vi "Create Database.vi"(8 "error in (no error)":errorcluster caption="entrée d'erreur (pas d'erreur)", 11 "Database Drivers en entrée":refnum<class "Database Drivers.lvclass">) -> (0 "error out":errorcluster caption="sortie d'erreur", 3 "Database Drivers en sortie":refnum<class "Database Drivers.lvclass">)   [LabVIEW 2020, in "Library Instrument & Equipement.lvlib" / "Library Database.lvlib" / "Database Drivers.lvclass"]
uses:
  Database Drivers.lvclass
  <vilib>/addons/database/Command.llb/Cmd Execute.vi
  <vilib>/addons/database/Recordset.llb/Rec Destroy - Command.vi
  <vilib>/addons/database/Command.llb/Cmd Delete.vi
  Database Drivers.lvclass/Database Drivers.ctl
  <vilib>/addons/database/NI_Database_API.lvlib
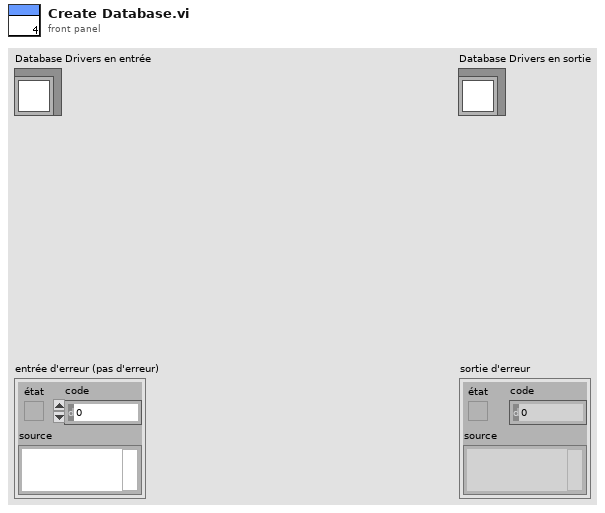
[diagram p1: front panel]
types:
  T1 = typedef "NI_Database_API.lvlib/Conn ObjectReference.ctl" = refnum<k1>
  T2 = typedef "NI_Database_API.lvlib/Cmd ObjectReference.ctl" = refnum<k1>
  T3 = typedef "NI_Database_API.lvlib/Cmd-Rec Object Reference.ctl" = refnum<k1>
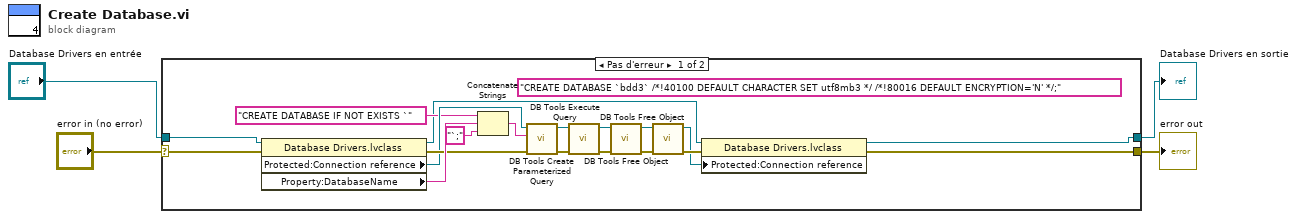
[diagram p0: block diagram]
diagram:
  n1 = case shown="Pas d'erreur" "error in (no error)" {
    selector: "error in (no error)" -> [w22 w25]
    tunnel: [w6 w25] -> w3
    tunnel: [w7 w24] -> w1
    tunnel: "Database Drivers en entrée" -> [w23 w24]
    frame No Error {
      (unwired) "CREATE DATABASE `bdd3` /*!40100 DEFAULT CHARACTER SET utf8mb3 */ /*!80016 DEFAULT ENCRYPTION='N' */;"
      n2 = property class="Database Drivers.lvclass"(reference=w23, error in=w22) -> (reference out=w8:refnum<class "Database Drivers.lvclass">, error out=w14:errorcluster, "Protected:Connection reference"=w11:T1, "Property:DatabaseName"=w16:string)
      n3 = Concatenate Strings("CREATE DATABASE IF NOT EXISTS `" ("chaîne"), w16, "`;" ("chaîne")) -> (w15:string)
      n4 = call <vilib>:"DB Tools Create Parameterized Query.vi"("error in (no error)"=w14, "SQL query"=w15, "connection reference"=w11) -> ("error out"=w21:errorcluster, "command reference"=w20:T2)  [unwired: 4 in, 1 out]
      n5 = call-poly <vilib>:"DB Tools Execute Query.vi"("error in (no error)"=w21, "command reference"=w20) -> ("error out"=w13:errorcluster, "command-recordset reference"=w18:T3)  [unwired: 6 in]
      n6 = call-poly <vilib>:"DB Tools Free Object.vi"("error in (no error)"=w13, "command-recordset reference"=w18) -> ("error out"=w12:errorcluster, "command reference"=w19:T2)  [unwired: 8 in]
      n7 = call-poly <vilib>:"DB Tools Free Object.vi"("error in (no error)"=w12, "command reference"=w19) -> ("error out"=w10:errorcluster, "connection reference"=w5:T1)  [unwired: 8 in]
      n8 = property class="Database Drivers.lvclass"(reference=w8, error in=w10, "Protected:Connection reference"=w5) -> (reference out=w7:refnum<class "Database Drivers.lvclass">, error out=w6:errorcluster)
    }
    frame Error {
    }
  }
  "error out" <- w3
  "Database Drivers en sortie" <- w1
